vi "update globals from init.vi"(1 "Manual Temp control":bool, 2 "Manual Power":dbl, 3 "Setpoint (C)":dbl=30.0, 7 "exp exec in":T2={"data file"={"autosave"=FALSE, "File refnum"=refnum, "data file path"=path ""}, "T log file"={"File refnum"=refnum, "T log file path"=path "", "exists"=FALSE}, "exp seq"={"wave params"={"Num of avg"=0, "Num points"=1000, "Meas rate (Hz)"=100000.0}, "Setpoints"=[], "#"=-1, "index"=-1, "elapsed time (s)"=0.0, "set time (s)"=0.0, "min settle (s)"=30.0, " Exec Status"=enum."Settling"}, "error"={"status"=FALSE, "code"=0, "source"=""}}, 11 "min set t":dbl caption="Min settle time (s)", 12 "exec.T mode":T1) -> (4 "Total elapsed time (s)":dbl=30.0, 8 "exp exec out":T2={"data file"={"autosave"=FALSE, "File refnum"=refnum, "data file path"=path ""}, "T log file"={"File refnum"=refnum, "T log file path"=path "", "exists"=FALSE}, "exp seq"={"wave params"={"Num of avg"=0, "Num points"=1000, "Meas rate (Hz)"=100000.0}, "Setpoints"=[], "#"=-1, "index"=-1, "elapsed time (s)"=0.0, "set time (s)"=0.0, "min settle (s)"=30.0, " Exec Status"=enum."Settling"}, "error"={"status"=FALSE, "code"=0, "source"=""}}, 13 "T params":T8={"Setpoint"=30.0, "Control Bandwidth"=4.0, "Integral Time"=30.0, "Int\nON"=TRUE, "Derivative Tme"=0.5, "Der\nON"=TRUE, "Settle Bandwidth"=1.0, "Settle Time"=30.0} {"Settle Time" step=1.0; "Settle Bandwidth" step=0.01; "Derivative Tme" step=0.01; "Integral Time" step=1.0; "Control Bandwidth" step=0.1; "Setpoint" step=0.1}, 14 "N Sets":i32 caption="Num of Setpoints", 15 "Setpoints":dbl[](array[numeric]) caption="Setpoint List")   [LabVIEW 2019]
doc: "This is a Bug C(T) subVI.\n\nThis subVI updates the bug global variables from the executive thread.\n\nPaul K Dixon\nP3600\nCSUSB Physics"
uses:
  typedefs/temp cont cluster.ctl
  typedefs/temp exec cluster.ctl
  typedefs/temp mode enum.ctl
  typedefs/temp indicator.ctl
  typedefs/temp control status.ctl
  typedefs/PID control parameters.ctl
  typedefs/temp cont utility.ctl
  typedefs/PID exec cluster.ctl
  typedefs/data file info.ctl
  typedefs/bug temp file info.ctl
  typedefs/exp seq cluster.ctl
  typedefs/wvfm acq params.ctl
  typedefs/bug meas status.ctl
  globals/Bug globals.vi
panel:
  out "T cont out":T9 {"utility"."therm volt" format="%_6g"; "utility"."heat volt in" format="%_6g"; "utility"."heat volt out" format="%_6g"; "utility"."power out" format="%_6g"; "utility"."H Vmax" format="%_6g"; "T exec"."man power" format="%_6g"; "T exec"."exec setpoint" format="%_6g"; "T params"."Settle Time" step=1.0; "T params"."Settle Bandwidth" step=0.01; "T params"."Derivative Tme" step=0.01; "T params"."Integral Time" step=1.0; "T params"."Control Bandwidth" step=0.1; "T params"."Setpoint" step=0.1; "T status"."Setpoint" format="%_6g"; "T status"."Power" format="%_6g"; "T status"."Temp" format="%_6g"}
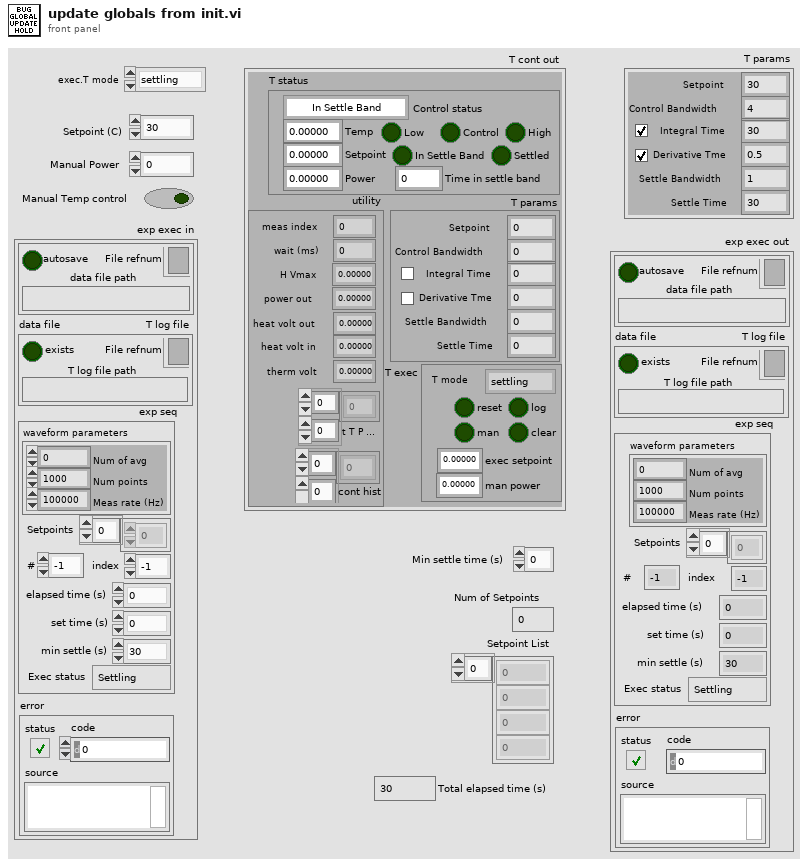
[diagram p1: front panel]
types:
  T1 = typedef "temp mode enum.ctl" = enum16{"settling", "measuring", "holding", "Exit"}
  T2 = typedef "PID exec cluster.ctl" = cluster{"data file":T3, "T log file":T4, "exp seq":T5, "error":errorcluster}
  T3 = typedef "data file info.ctl" = cluster{"autosave":bool, "File refnum":refnum<file>, "data file path":path}
  T4 = typedef "bug temp file info.ctl" = cluster{"File refnum":refnum<file>, "T log file path":path, "exists":bool}
  T5 = typedef "exp seq cluster.ctl" = cluster{"wave params":T6, "Setpoints":dbl[], "#":i32, "index":i32, "elapsed time (s)":dbl, "set time (s)":dbl, "min settle (s)":dbl, " Exec Status":T7}
  T6 = typedef "wvfm acq params.ctl" = cluster{"Num of avg":i32, "Num points":i32, "Meas rate (Hz)":dbl}
  T7 = typedef "bug meas status.ctl" = enum32{"Settling", "Measuring", "Holding", "Exit"}
  T8 = typedef "PID control parameters.ctl" = cluster{"Setpoint":dbl, "Control Bandwidth":dbl, "Integral Time":dbl, "Int\nON":bool, "Derivative Tme":dbl, "Der\nON":bool, "Settle Bandwidth":dbl, "Settle Time":dbl}
  T9 = typedef "temp cont cluster.ctl" = cluster{"T exec":T10, "T status":T11, "T params":T8, "utility":T13}
  T10 = typedef "temp exec cluster.ctl" = cluster{"T mode":T1, "exec setpoint":dbl, "reset":bool, "man power":dbl, "man":bool, "log":bool, "clear":bool}
  T11 = typedef "temp indicator.ctl" = cluster{"Control status":T12, "Temp":dbl, "Power":dbl, "Time in settle band":dbl, "Settled":bool, "Low":bool, "High":bool, "Setpoint":dbl, "Control":bool, "In Settle Band":bool}
  T12 = typedef "temp control status.ctl" = enum16{"In Settle Band", "In Control Band", "Below Control Band", "Above Control Band"}
  T13 = typedef "temp cont utility.ctl" = cluster{"meas index":i32, "wait (ms)":i32, "H Vmax":dbl, "power out":dbl, "heat volt out":dbl, "heat volt in":dbl, "therm volt":dbl, "t T P hist":dbl[][], "cont hist":dbl[][]}
  T14 = typedef "measurement.ctl" = cluster{"wvfm params":T6, "avg":waveform(dbl), "raw wvfms":waveform(dbl)[], "progress":cluster{"avg done":bool, "meas index":i32, "N waves":i32}, "t (s)":dbl}
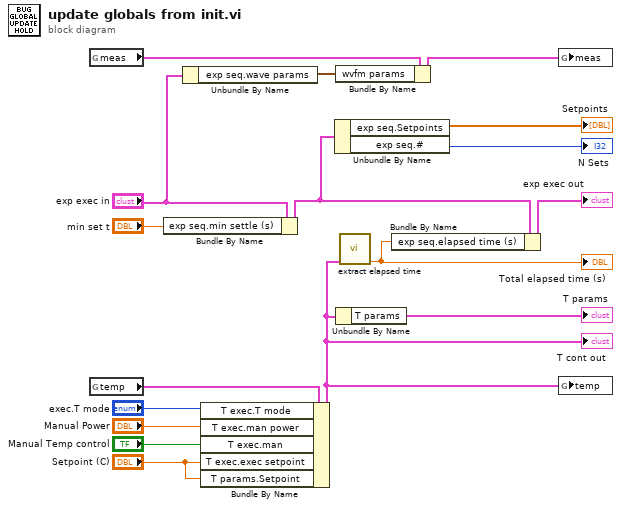
[diagram p0: block diagram]
diagram:
  n1 = global read "Bug globals.vi" "meas"() -> (w5:T14)
  n2 = global read "Bug globals.vi" "temp"() -> (w14:T9)
  n3 = Bundle By Name(cluster="exp exec in", "exp seq.min settle (s)"="min set t") -> (w8:T2)
  n4 = Unbundle By Name("exp exec in") -> ("exp seq.wave params"=w3:T6)
  n5 = Bundle By Name(cluster=w14, "T exec.T mode"="exec.T mode", "T exec.man power"="Manual Power", "T exec.man"="Manual Temp control", "T exec.exec setpoint"="Setpoint (C)", "T params.Setpoint"="Setpoint (C)") -> (w2:T9)
  "T cont out" <- w2
  n6 = Unbundle By Name(w8) -> ("exp seq.Setpoints"=→"Setpoints":dbl[], "exp seq.#"=→"N Sets":i32)
  n7 = Bundle By Name(cluster=w5, "wvfm params"=w3) -> (w4:T14)
  n8 = Unbundle By Name(w2) -> ("T params"=→"T params":T8)
  n9 = call "extract elapsed time.vi"("temp"=w2) -> ("latest time (s)"=w1:dbl)  [unwired: 14 in]
  "Total elapsed time (s)" <- w1
  n10 = Bundle By Name(cluster=w8, "exp seq.elapsed time (s)"=w1) -> (→"exp exec out":T2)
  n11 = global write "Bug globals.vi" "meas"(w4) -> ()
  n12 = global write "Bug globals.vi" "temp"(w2) -> ()
